vi "Event Structure in Empty Space Equivalent.vi"   [LabVIEW 2017]
uses:
  <vilib>/Utility/inputDevices.llb/mouseAcquire.vi
  <vilib>/Utility/inputDevices.llb/closeMouse.vi
types:
  T1 = cluster{"button 1":bool, "button 2":bool, "button 3":bool, "button 4":bool}
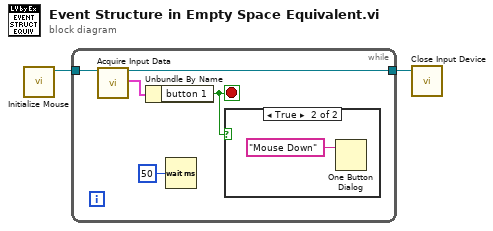
[diagram p0: block diagram]
diagram:
  n1 = call <vilib>:"Initialize Mouse.vi"() -> ("device ID"=w2:refnum<k1>)  [unwired: 10 in, 1 out]
  n2 = while {
    tunnel: w2 -> [w7]
    tunnel: [w4] -> w1
    stop <- w5 stop-if-true
    n3 = call-poly <vilib>:"Acquire Input Data.vi"("device ID"=w7) -> ("device ID"=w4:refnum<k1>, "button info"=w6:T1)  [unwired: 15 in, 2 out]
    n4 = Unbundle By Name(w6) -> ("button 1"=w5:bool)
    n5 = Wait (ms)(milliseconds to wait=u32 50) -> ()  [unwired: 1 out]
    n6 = case shown="True" w5 {
      frame False {
      }
      frame True {
        n7 = One Button Dialog(message="Mouse Down") -> ()  [unwired: 1 in, 1 out]
      }
    }
  }
  n8 = call-poly <vilib>:"Close Input Device.vi"("device ID"=w1) -> ()  [unwired: 9 in, 1 out]
